vi "Distance Sensor PWM TEST.vi"() -> ()   [LabVIEW 2017]
doc: "This example shows how to use the MaxBotix LV-MaxSonar-EZ1 Sonar Range Finder MB1010. It will display the distance from the sensor in inches.\n\nThis example expects a USB cable connected from your development PC to the Type B USB Jack (next to the power input) on the roboRIO."
uses:
  <vilib>/Rock Robotics/SystemInterfaces/DIO/FPGA_DIOChannel.ctl
panel:
  in  "Max Distance":dbl=52.0
  in  "Min Distance":dbl=1.0
  in  "PWM Frequency":dbl=245.0
  out "distance":dbl(slide)=125.0 scale=0.0..100.0 scale format="%3d"
  in  "DIO Channel":T1
  in  "stop":bool
  # "Set these inputs before running."
  # "inches"
  # "Output information."
  # "EZ1"
  # "GND (black wire)------\n+5 (red wire)----------\nPW (white wire)-------"
  # "roboRIO\nDIO-5 \nDIO-5  V\nDIO-5  S"
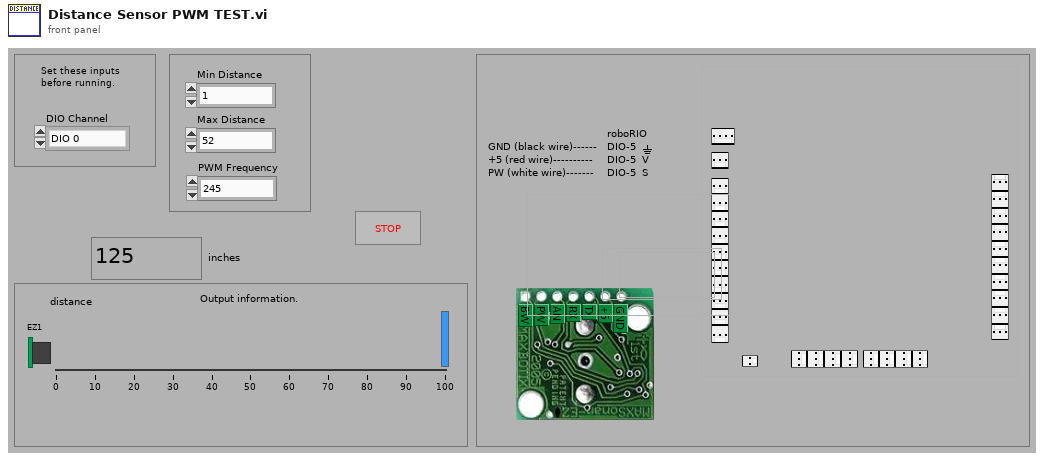
[diagram p1: front panel]
types:
  T1 = typedef "FPGA_DIOChannel.ctl" = enum8{"DIO 0", "DIO 1", "DIO 2", "DIO 3", "DIO 4", "DIO 5", "DIO 6", "DIO 7", "DIO 8", "DIO 9", "DIO MXP 0", "DIO MXP 1", "DIO MXP 2", "DIO MXP 3", "DIO MXP 4", "DIO MXP 5", "DIO MXP 6", "DIO MXP 7", "DIO MXP 8", "DIO MXP 9", "DIO MXP 10", "DIO MXP 11", "DIO MXP 12", "DIO MXP 13", "DIO MXP 14", "DIO MXP 15", "SPI Port CS1", "SPI Port CS2", "SPI Port CS3", "SPI Port MISO", "SPI Port MOSI", "Invalid"}
  T2 = typedef "Cluster_Distance PWM Reference.ctl" = cluster{"CounterDevRef":T3, "Min Distance":dbl, "Max Distance":dbl, "PWM Frequency":dbl, "DIO Channel":T1}
  T3 = typedef "WPI_CounterDevRef.ctl" = cluster{"DevStatus":errorcluster, "CntIndex":T4}
  T4 = typedef "FPGA_CounterCtrSystemIndex.ctl" = enum8{"Ctr 0", "Ctr 1", "Ctr 2", "Ctr 3", "Ctr 4", "Ctr 5", "Ctr 6", "Ctr 7", "Invalid"}
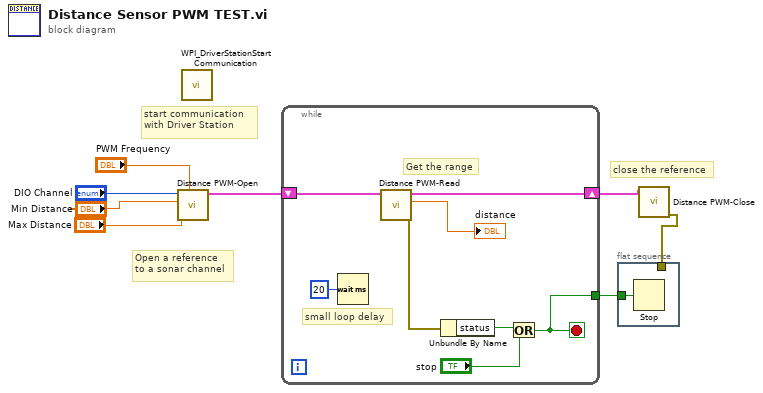
[diagram p0: block diagram]
diagram:
  # "start communication with Driver Station"
  # "close the reference"
  # "Open a reference\nto a sonar channel"
  n1 = call "Distance PWM-Open.vi"("PWM Frequency"="PWM Frequency", "Max Distance"="Max Distance", "Min Distance"="Min Distance", "DIO Channel"="DIO Channel") -> ("Distance PWM Ref"=w3:T2)  [unwired: 6 in, 1 out]
  n2 = call <vilib>:"WPI_DriverStationStart Communication.vi"() -> ()  [unwired: 2 in, 10 out]
  n3 = while {
    shift-right: [w9] -> w1
    shift-left: w3 -> [w10]
    tunnel: [w14] -> w8
    stop <- w14 stop-if-true
    # "small loop delay"
    # "Get the range"
    n4 = Wait (ms)(milliseconds to wait=u32 20) -> ()  [unwired: 1 out]
    n5 = call "Distance PWM-Read.vi"("SonarMB1010DigitalDevRef"=w10) -> ("Error Out"=w13:errorcluster, "Distance Out"=→"distance":dbl, "SonarMB1010DigitalDevRef Out"=w9:T2)  [unwired: 8 in]
    n6 = Unbundle By Name(w13) -> ("status"=w15:bool)
    n7 = Or(x=w15, y="stop") -> (x .or. y?=w14:bool)
  }
  n8 = flat-sequence {
    tunnel: w8 -> [w17]
    tunnel: w2 -> [_]
    frame #0 {
      n9 = Stop(stop? (T)=w17) -> ()
    }
  }
  n10 = call "Distance PWM-Close.vi"("SonarMB1010DigitalDevRef"=w1) -> ("Error Out"=w2:errorcluster)  [unwired: 10 in]
